vi "Set Manifold Port.vi"(8 "error in":errorcluster, 9 "On/Off":bool, 10 "Manifold Port":i32, 11 "Gantry in":refnum<class "Gantry.lvclass">) -> (0 "error out":errorcluster, 3 "Gantry out":refnum<class "Gantry.lvclass">)   [LabVIEW 2026, in "Gantry.lvclass"]
uses:
  Gantry.lvclass
  <vilib>/DAQmx/miscellaneous.llb/DAQmx Fill In Error Info.vi
  FlexWorktable/FlexWorktable.lvclass
  Gantry.lvclass/Gantry.ctl
  <vilib>/DAQmx/write.llb/DAQmx Write (Digital 1D Bool NChan 1Samp 1Line).vi
  GH2/GH2.lvclass
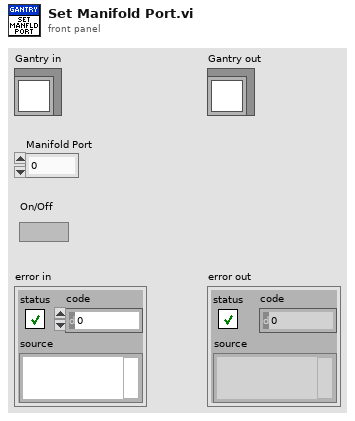
[diagram p1: front panel]
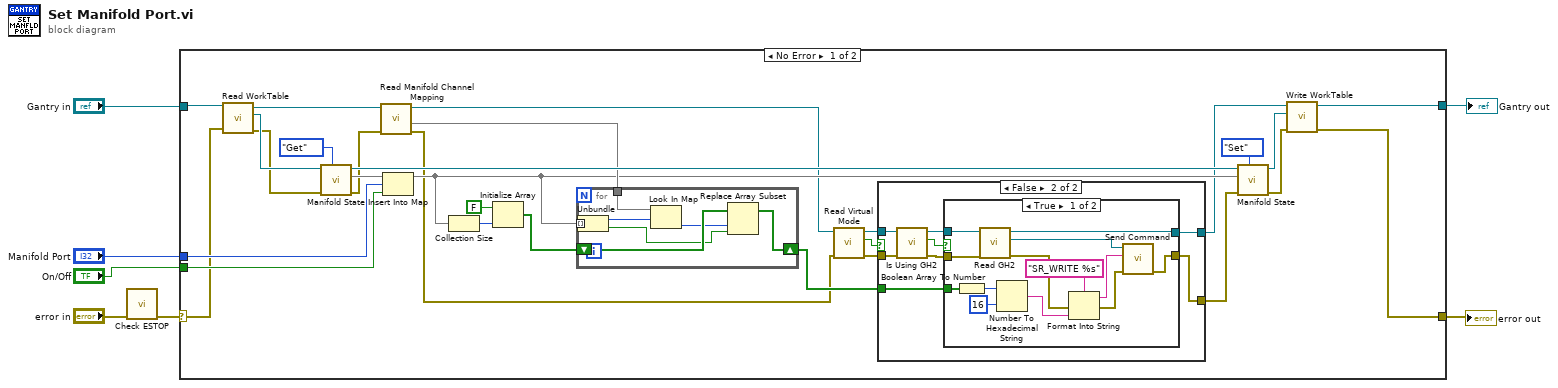
[diagram p0: block diagram]
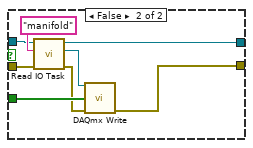
[diagram p3: hidden frame]
diagram:
  n1 = call "Check ESTOP.vi"("error in"="error in") -> ("error out"=w2:errorcluster)  [unwired: 10 in]
  n2 = case shown="No Error" w2 {
    selector: w2 -> [w14 w76]
    tunnel: [w18 w76] -> w7
    tunnel: [w19 w75] -> w6
    tunnel: "Gantry in" -> [w15 w75]
    tunnel: "Manifold Port" -> [w28 _]
    tunnel: "On/Off" -> [w27 _]
    frame No Error {
      n3 = call-dynamic "Read WorkTable.vi"("error in"=w14, "Gantry Class in"=w15) -> ("error out"=w16:errorcluster, "Worktable"=w32:refnum<class "FlexWorktable.lvclass">, "Gantry Class out"=w17:refnum<class "Gantry.lvclass">)  [unwired: 7 in]
      n4 = call-dynamic "Manifold State.vi"("Get/Set"=enum16{"Get", "Set"}."Get", "error in (no error)"=w16, "FlexWorktable in"=w32) -> ("error out"=w26:errorcluster, "Port Statuses"=w29:map{i32, bool}, "FlexWorktable out"=w35:refnum<class "FlexWorktable.lvclass">)  [unwired: 6 in]
      n5 = call "Read Manifold Channel Mapping.vi"("error in (no error)"=w26, "Gantry in"=w17) -> ("error out"=w11:errorcluster, "Port -> Channel"=w25:map{i32, i32}, "Gantry out"=w13:refnum<class "Gantry.lvclass">)  [unwired: 6 in, 1 out]
      n6 = Insert Into Map(map in=w29, key=w28, value=w27) -> (map out=w24:map{i32, bool})  [unwired: 2 out]
      n7 = Collection Size(1:w24) -> (0:w23:i32)
      n8 = Initialize Array(FALSE, w23) -> (w21:bool[])
      n9 = for {
        tunnel: w24 -> [w43] mode=indexing
        tunnel: w25 -> [w42]
        shift-right: [w39] -> w20
        shift-left: w21 -> [w40]
        n10 = Unbundle(w43) -> (w41:i32, w37:bool)
        n11 = Look In Map(map=w42, key=w41) -> (value=w38:i32)  [unwired: 1 in, 1 out]
        n12 = Replace Array Subset(array=w40, new element=w37, index=w38) -> (w39:bool[])
      }
      n13 = call-dynamic "Read Virtual Mode.vi"("error in (no error)"=w11, "Gantry in"=w13) -> ("error out"=w10:errorcluster, "Is Virtual"=w9:bool, "Gantry out"=w12:refnum<class "Gantry.lvclass">)  [unwired: 6 in, 1 out]
      n14 = case shown="False" w9 {
        tunnel: [w45 w53] -> w33
        tunnel: w20 -> [_ w52]
        tunnel: w10 -> [w45 w51]
        tunnel: w12 -> [w44 w47]
        tunnel: [w44 w46] -> w8
        frame True {
        }
        frame False {
          n15 = call "Is Using GH2.vi"("error in (no error)"=w51, "Gantry in"=w47) -> ("error out"=w48:errorcluster, "Using GH2"=w49:bool, "Gantry out"=w50:refnum<class "Gantry.lvclass">)  [unwired: 7 in]
          n16 = case shown="True" w49 {
            tunnel: [w62 w74] -> w53
            tunnel: w52 -> [w61 w73]
            tunnel: w50 -> [w66 w70]
            tunnel: w48 -> [w64 w71]
            tunnel: [w65 w68] -> w46
            frame True {
              n17 = Boolean Array To Number(Boolean array=w61) -> (number=w60:u32)
              n18 = call "Read GH2.vi"("error in (no error)"=w64, "Gantry in"=w66) -> ("error out"=w58:errorcluster, "GH2.lvclass"=w63:refnum<class "GH2.lvclass">, "Gantry out"=w65:refnum<class "Gantry.lvclass">)  [unwired: 7 in]
              n19 = Number To Hexadecimal String(1:i16 16 ("width (-)"), 2:w60) -> (0:w54:string)
              n20 = Format Into String(format string="SR_WRITE %s", error in=w58, w54) -> (resulting string=w56:string, error out=w57:errorcluster)  [unwired: 1 in]
              n21 = call "Send Command.vi"("error in (no error)"=w57, "command"=w56, "GH2 in"=w63) -> ("error out"=w62:errorcluster)  [unwired: 6 in, 2 out]
            }
            frame False {
              n22 = call "Read IO Task.vi"("error in (no error)"=w71, "Task Name"="manifold", "Gantry in"=w70) -> ("error out"=w67:errorcluster, "task/channels in"=w69:refnum<k21>, "Gantry out"=w68:refnum<class "Gantry.lvclass">)  [unwired: 6 in]
              n23 = call-poly <vilib>:"DAQmx Write.vi"("task/channels in"=w69, "data"=w73, "error in"=w67) -> ("error out"=w74:errorcluster)  [unwired: 10 in, 2 out]
            }
          }
        }
      }
      n24 = call-dynamic "Manifold State.vi"("Get/Set"=enum16{"Get", "Set"}."Set", "error in (no error)"=w33, "New Port Statuses"=w24, "FlexWorktable in"=w35) -> ("error out"=w30:errorcluster, "FlexWorktable out"=w31:refnum<class "FlexWorktable.lvclass">)  [unwired: 5 in, 1 out]
      n25 = call-dynamic "Write WorkTable.vi"("error in (no error)"=w30, "FlexWorktable"=w31, "Gantry Class in"=w8) -> ("error out"=w18:errorcluster, "Gantry Class out"=w19:refnum<class "Gantry.lvclass">)  [unwired: 7 in]
    }
    frame Error {
    }
  }
  "error out" <- w7
  "Gantry out" <- w6
